vi "test 03 - DIM.vi"() -> ()   [LabVIEW 2020]
uses:
  UI_Actor/UI_Actor/ctl_AR_Parameters.ctl
  UI_Actor/UI_Actor/ctl_AR_Mode.ctl
  support/Databox.lvlibp/TypesTools/Config/Config.lvclass
  support/Databox.lvlibp/TypesTools/Data/Data.lvclass
  support/Databox.lvlibp/TypesTools/Data/TypeEnum.ctl
  UIA_UTsupport/UIA_UTsupport.lvclass
  D:/Projets/STEP AT/UI Actor/UI_Actor/UI_Actor/UI_Actor.lvclass
  UI_Actor/UI_Actor Messages/UI_AutoRefresh Msg/UI_AutoRefresh Msg.lvclass/UI_AutoRefresh Msg.ctl
  support/Actor Framework.lvlibp/Message Enqueuer/Enqueue.vi
  UIA_UTsupport/gloglo.vi
  UI_Actor/UI_Actor Messages/UI_AutoRefresh Msg/UI_AutoRefresh Msg.lvclass
  UI_Actor/UI_Actor/UI_Actor.lvclass
  support/Actor Framework.lvlibp/Stop Msg/Stop Msg.lvclass
panel:
  out "Latest Data":dbl[](array[numeric])
  out "DIM SysLabels":string[](array[string])
  out "PASS":bool
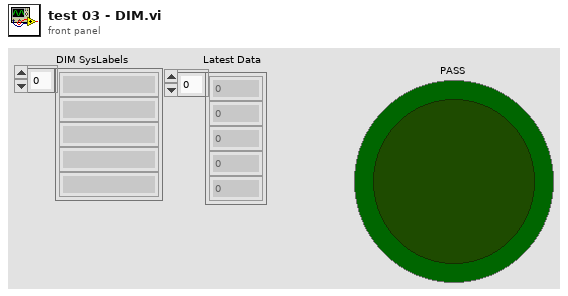
[diagram p1: front panel]
types:
  T1 = typedef "Databox.lvlibp/Data.lvclass/TypeEnum.ctl" = enum16{"Boolean", "SByte", "Byte", "Int16", "UInt16", "Int32", "UInt32", "Int64", "UInt64", "Float", "Double", "String", "DateTime", "ByteString", "Array of Boolean", "Array of SByte", "Array of Byte", "Array of Int16", "Array of UInt16", "Array of Int32", "Array of UInt32", "Array of Int64", "Array of UInt64", "Array of Float", "Array of Double", "Array of String", "Array of DateTime", "Array of ByteString", "Matrix of Boolean", "Matrix of SByte", "Matrix of Byte", "Matrix of Int16", "Matrix of UInt16", "Matrix of Int32", "Matrix of UInt32", "Matrix of Int64", "Matrix of UInt64", "Matrix of Float", "Matrix of Double", "Matrix of String ", "Matrix of DateTime", "Matrix of ByteString"}
  T2 = cluster{"Ch.Conf":refnum<class "Config.lvclass">, "Data":refnum<class "Data.lvclass">[]}
  T3 = typedef "UI_Actor.lvlib/UI_Actor.lvclass/ctl_AR_Parameters.ctl" = cluster{"Write TipStrips with details (T)":bool, "Write Captions with UserLabels (T)":bool, "Mode (ind only)":T4, "Enable nested stream (T)":bool}
  T4 = typedef "UI_Actor.lvlib/UI_Actor.lvclass/ctl_AR_Mode.ctl" = enum16{"Controls only", "Indicators only", "All"}
  T5 = cluster{"Ch.Conf":refnum<class "Config.lvclass">, "Data":refnum<class "Data.lvclass">[]}[]
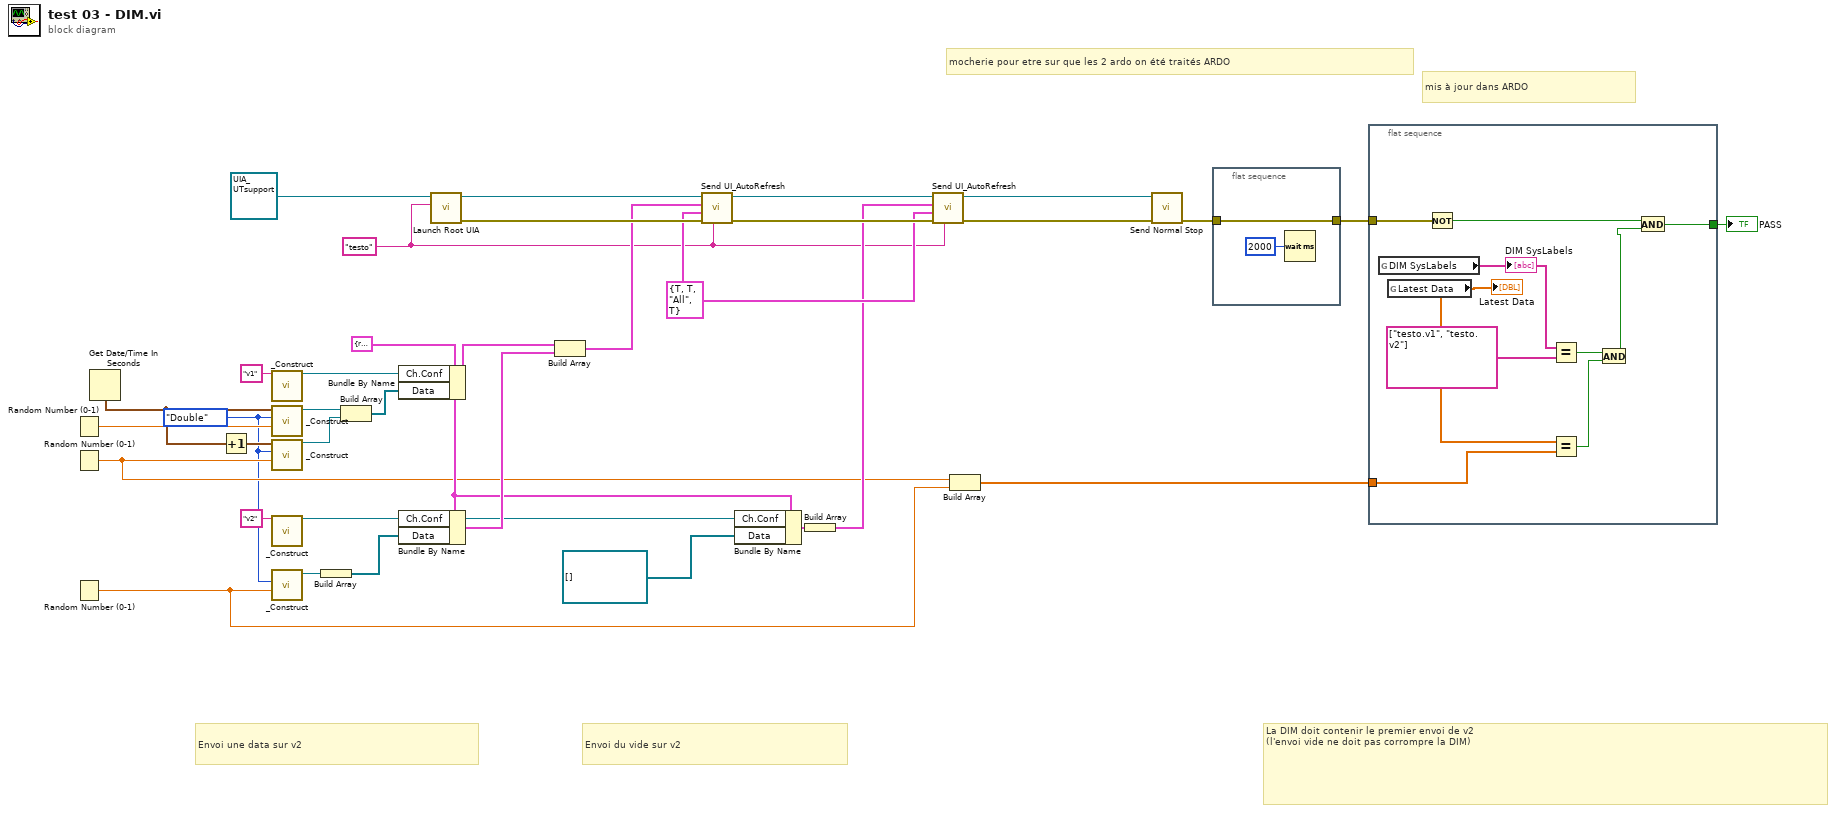
[diagram p0: block diagram]
diagram:
  w4 = TypeEnum."Double" ("Type")
  w10 = T2 {"Ch.Conf"=refnum, "Data"=[]} ("Cluster")
  w2 = "testo" ("Actor Name")
  w17 = T3 {"Write TipStrips with details (T)"=TRUE, "Write Captions with UserLabels (T)"=TRUE, "Mode (ind only)"=enum."All", "Enable nested stream (T)"=TRUE} ("Parameters (Tipstrips,Captions,All)")
  # "mocherie pour etre sur que les 2 ardo on été traités ARDO"
  # "mis à jour dans ARDO"
  # "La DIM doit contenir le premier envoi de v2\n(l'envoi vide ne doit pas corrompre la DIM)"
  # "Envoi du vide sur v2"
  # "Envoi une data sur v2"
  n1 = Random Number (0-1)() -> (number: 0 to 1=w14:dbl)
  n2 = Random Number (0-1)() -> (number: 0 to 1=w5:dbl)
  n3 = Random Number (0-1)() -> (number: 0 to 1=w3:dbl)
  n4 = Get Date/Time In Seconds() -> (seconds since 1Jan1904=w16:timestamp)
  n5 = Increment(x=w16) -> (x+1=w15:timestamp)
  n6 = call "_Construct.vi"("System Label"="v1") -> ("Ch.Conf out"=w32:refnum<class "Config.lvclass">)  [unwired: 13 in, 1 out]
  n7 = call "_Construct.vi"("Value"=w14, "Type"=w4, "Time (now!)"=w16) -> ("Ch.TData out"=w30:refnum<class "Data.lvclass">)  [unwired: 7 in, 1 out]
  n8 = call "_Construct.vi"("Value"=w5, "Type"=w4, "Time (now!)"=w15) -> ("Ch.TData out"=w29:refnum<class "Data.lvclass">)  [unwired: 7 in, 1 out]
  n9 = call "_Construct.vi"("System Label"="v2") -> ("Ch.Conf out"=w11:refnum<class "Config.lvclass">)  [unwired: 13 in, 1 out]
  n10 = call "_Construct.vi"("Value"=w3, "Type"=w4) -> ("Ch.TData out"=w7:refnum<class "Data.lvclass">)  [unwired: 8 in, 1 out]
  n11 = Build Array(w7) -> (w6:refnum<class "Data.lvclass">[])
  n12 = Build Array(w30, w29) -> (w28:refnum<class "Data.lvclass">[])
  n13 = Bundle By Name(cluster=w10, "Ch.Conf"=w32, "Data"=w28) -> (w33:T2)
  n14 = Bundle By Name(cluster=w10, "Ch.Conf"=w11, "Data"=w6) -> (w31:T2)
  n15 = call "Launch Root UIA.vi"("Actor Name"=w2, "UI_Actor in"=refnum<class "UIA_UTsupport.lvclass"> refnum ("UIA_UTsupport.lvlib:UIA_UTsupport.lvclass")) -> ("error out"=w35:errorcluster, "Actor's Enqueuer"=w25:refnum<class "Message Enqueuer.lvclass">)  [unwired: 8 in]
  n16 = Build Array(w33, w31) -> (w34:T5)
  n17 = call "Send UI_AutoRefresh.vi"("Sourcer name"=w2, "error in (no error)"=w35, "Parameters (Tipstrips,Captions,All)"=w17, "Data chunk"=w34, "Message Enqueuer"=w25) -> ("error out"=w20:errorcluster, "Message Enqueuer out"=w21:refnum<class "Message Enqueuer.lvclass">)  [unwired: 5 in]
  n18 = Bundle By Name(cluster=w10, "Ch.Conf"=w11, "Data"=refnum<class "Data.lvclass">[] []) -> (w9:T2)
  n19 = Build Array(w9) -> (w8:T5)
  n20 = call "Send UI_AutoRefresh.vi"("Sourcer name"=w2, "error in (no error)"=w20, "Parameters (Tipstrips,Captions,All)"=w17, "Data chunk"=w8, "Message Enqueuer"=w21) -> ("error out"=w19:errorcluster, "Message Enqueuer out"=w18:refnum<class "Message Enqueuer.lvclass">)  [unwired: 5 in]
  n21 = Build Array(w5, w3) -> (w13:dbl[])
  n22 = call "Send Normal Stop.vi"("error in (no error)"=w19, "Message Enqueuer"=w18) -> ("error out"=w23:errorcluster)  [unwired: 9 in]
  n23 = flat-sequence {
    tunnel: w23 -> [w36]
    tunnel: [w36] -> w22
    frame #0 {
      n24 = Wait (ms)(milliseconds to wait=u32 2000) -> ()  [unwired: 1 out]
    }
  }
  n25 = flat-sequence {
    tunnel: w22 -> [w47]
    tunnel: [w45] -> w24
    tunnel: w13 -> [w42]
    frame #0 {
      n26 = global read "gloglo.vi" "DIM SysLabels"() -> (w39:string[])
      "DIM SysLabels" <- w39
      n27 = global read "gloglo.vi" "Latest Data"() -> (w38:dbl[])
      "Latest Data" <- w38
      n28 = Not(x=w47) -> (.not. x?=w46:bool)
      n29 = Equal?(x=w39, y=string[] ["testo.v1", "testo.v2"] ("DIM SysLabels")) -> (x = y?=w43:bool)
      n30 = Equal?(x=w38, y=w42) -> (x = y?=w41:bool)
      n31 = And(x=w43, y=w41) -> (x .and. y?=w40:bool)
      n32 = And(x=w46, y=w40) -> (x .and. y?=w45:bool)
    }
  }
  "PASS" <- w24
